vi "manipulator_command.vi"(8 "Error in":errorcluster, 9 "Manipulator command":sgl[](array[numeric]), 11 "Micron config":T1) -> (0 "Error out":errorcluster)   [LabVIEW 2014]
uses:
  initialization/micron_config.ctl
  i2c_interface.ctl
  fpga_reference.ctl
  testing/Micron params.ctl
  testing/stimulus.ctl
  testing/injection_point.ctl
  filtering/goal_loop_parms.ctl
  testing/mode_conrols.ctl
  testing/manipulator_cal.ctl
  asap/labview/testing/probe_calibration.ctl
  host/network_params.ctl
  cancellation/sq_control_params.ctl
  cancellation/decoupled_gain.ctl
  cancellation/estimation_controls.ctl
panel:
  # "This VI writes out the manipulator command, with appropriate \nscaling and limit checking."
  # "This is a somewhat arbitrary tuning parameter.  The nominal value according to the nominal motor resonant freq is 171 kHz/Fs = 170, but different values may give better results.  A modestly inflated value helps to insure that we can drive the motor to 100% duty."
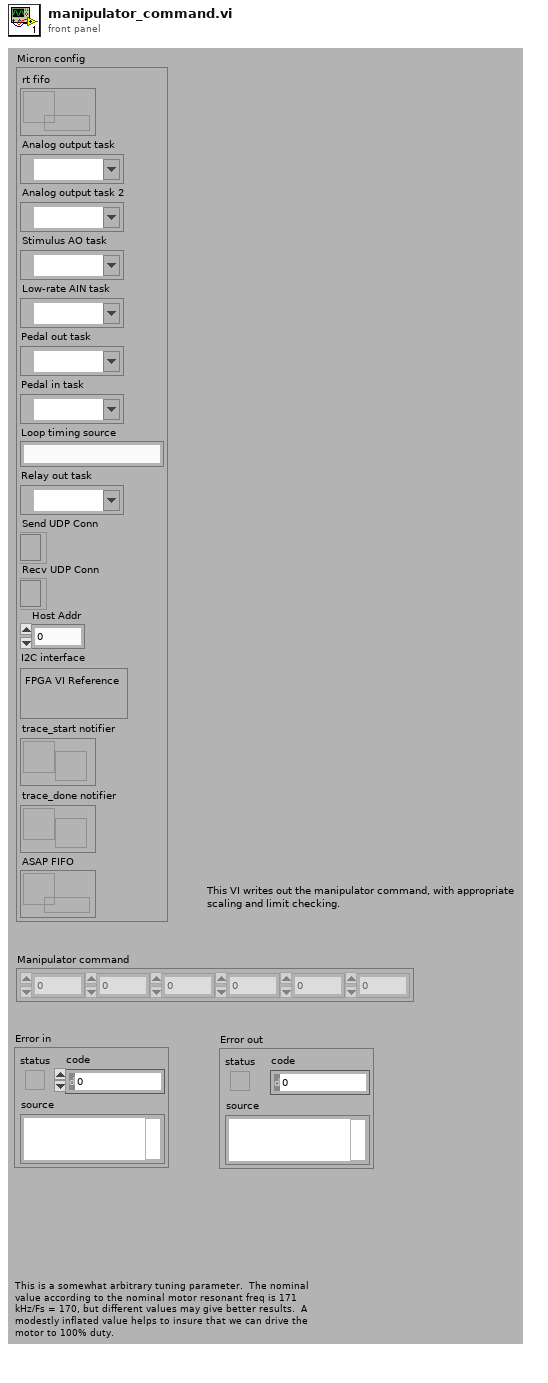
[diagram p1: front panel]
types:
  T1 = typedef "micron_config.ctl" = cluster{"rt fifo":refnum<k33>, "Analog output task":refnum<k21>, "Analog output task 2":refnum<k21>, "Stimulus AO task":refnum<k21>, "Low-rate AIN task":refnum<k21>, "Pedal out task":refnum<k21>, "Pedal in task":refnum<k21>, "Loop timing source":string, "Relay out task":refnum<k21>, "Send UDP Conn":refnum<k16>, "Recv UDP Conn":refnum<k16>, "Host Addr":u32, "I2C interface":T2, "trace_start notifier":refnum<notifier>, "trace_done notifier":refnum<notifier>, "ASAP FIFO":refnum<k33>}
  T2 = typedef "i2c_interface.ctl" = cluster{"FPGA VI Reference":T3}
  T3 = typedef "fpga_reference.ctl" = refnum<k20>
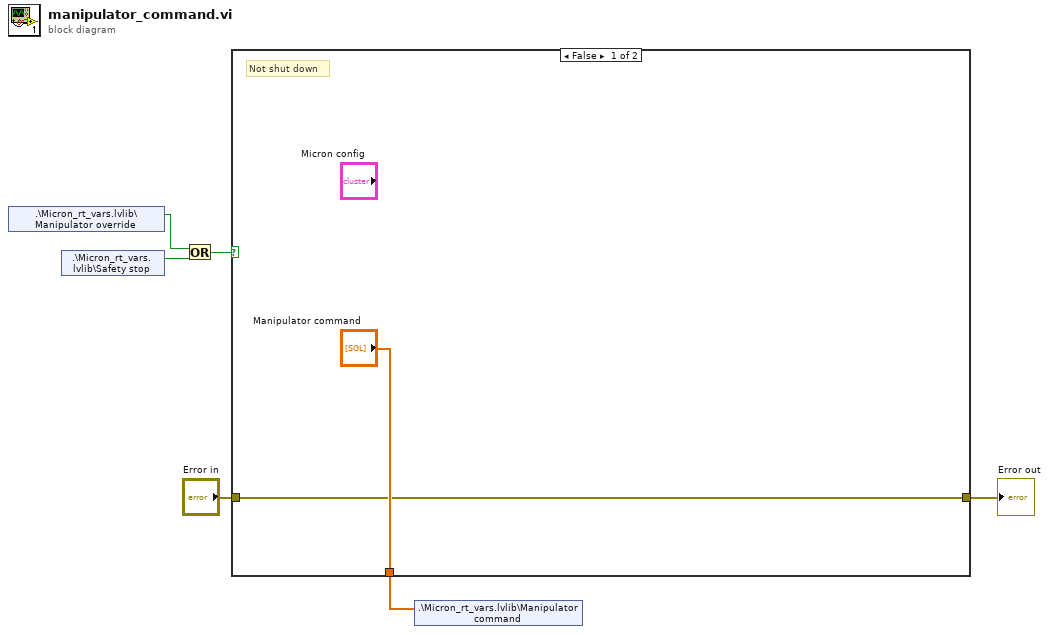
[diagram p0: block diagram]
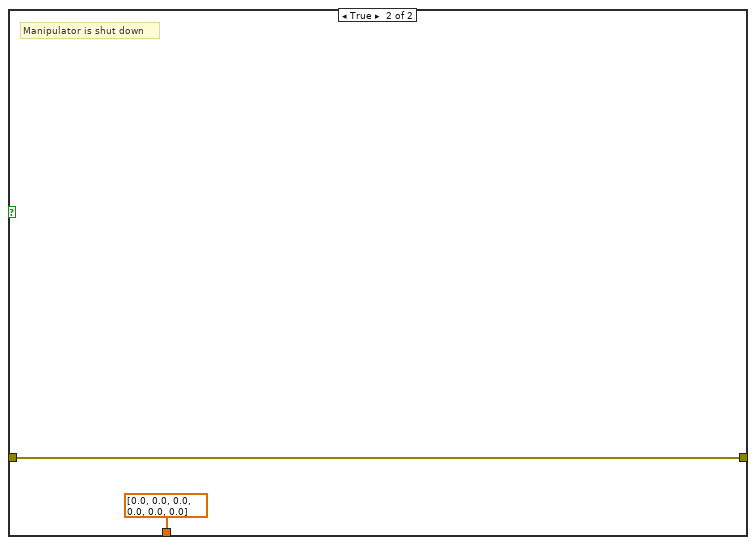
[diagram p2: hidden frame]
diagram:
  n1 = shared-variable ".\\Micron_rt_vars.lvlib\\Manipulator override"() -> (w3:bool)  [unwired: 1 in, 1 out]
  n2 = shared-variable ".\\Micron_rt_vars.lvlib\\Safety stop"() -> (w4:bool)  [unwired: 1 in, 1 out]
  n3 = Or(x=w3, y=w4) -> (x .or. y?=w2:bool)
  n4 = case shown="False" w2 {
    tunnel: "Error in" -> [w7 w10]
    tunnel: [w7 w10] -> w5
    tunnel: ["Manipulator command" sgl[] [0.0, 0.0, 0.0, 0.0, 0.0, 0.0] ("Manipulator command")] -> w1
    frame False {
      # "Not shut down"
    }
    frame True {
      # "Manipulator is shut down"
    }
  }
  "Error out" <- w5
  n5 = shared-variable ".\\Micron_rt_vars.lvlib\\Manipulator command"(w1) -> ()  [unwired: 1 in, 1 out]
